vi "ArrayFirst_I.vi"(11 "1D Array In":i32[](array[numeric])) -> (2 "Rest of Array":i32[](array[numeric]), 3 "First Element":i32)   [LabVIEW 2013]
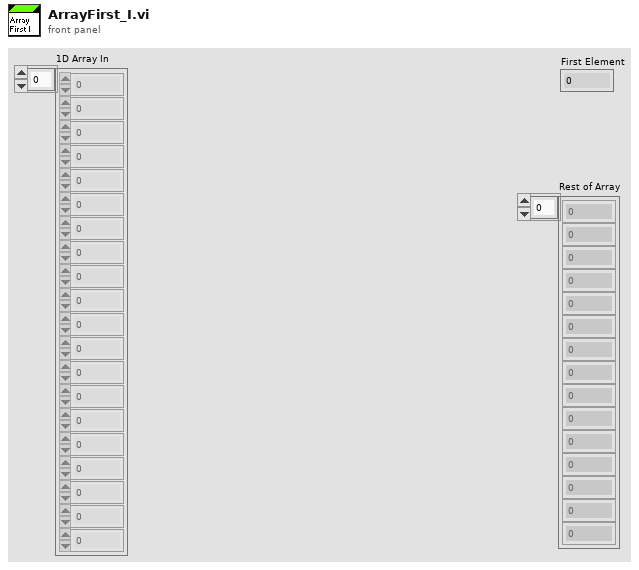
[diagram p1: front panel]
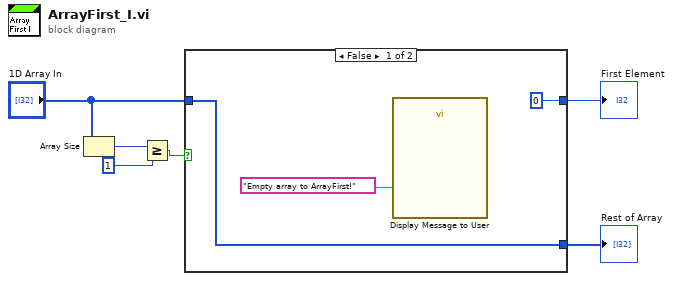
[diagram p0: block diagram]
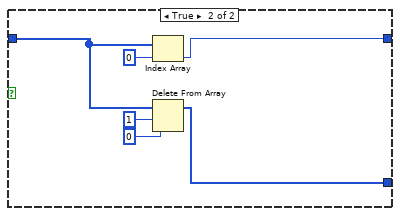
[diagram p2: hidden frame]
diagram:
  n1 = Array Size(array="1D Array In") -> (size(s)=w6:i32)
  n2 = Greater Or Equal?(x=w6, y=1) -> (x >= y?=w4:bool)
  n3 = case shown="False" w4 {
    tunnel: "1D Array In" -> [w8 w11]
    tunnel: [0 ("Numeric") w14] -> w2
    tunnel: [w8 w10] -> w1
    frame False {
      n4 = call "Display Message to User"("Message"="Empty array to ArrayFirst!") -> ()  [unwired: 9 in, 2 out]
    }
    frame True {
      n5 = Index Array(array=w11, index=0) -> (element=w14:i32)
      n6 = Delete From Array(array=w11, length=1, index=0) -> (array with subset deleted=w10:i32[])  [unwired: 1 out]
    }
  }
  "First Element" <- w2
  "Rest of Array" <- w1
